vi "首页设置.vi"() -> ()   [LabVIEW 2016]
uses:
  <vilib>/Utility/config.llb/NI_LVConfig.lvlib
panel:
  in  "关闭":bool
  in  "底部状态栏显示信息":string="一体化微型水质监测系统"
  in  "流速":bool caption="氨氮禁用"
  in  "瞬时流量":bool caption="氨氮禁用"
  in  "湿度":bool=TRUE caption="氨氮禁用"
  in  "水位":bool caption="氨氮禁用"
  in  "室温":bool=TRUE caption="氨氮禁用"
  in  "CODCr":bool caption="氨氮禁用"
  in  "CODMn":bool caption="氨氮禁用"
  in  "总氮":bool caption="氨氮禁用"
  in  "总磷":bool caption="氨氮禁用"
  in  "氨氮":bool caption="氨氮禁用"
  in  "Turb":bool caption="氨氮禁用"
  in  "Cond":bool caption="氨氮禁用"
  in  "DO":bool caption="氨氮禁用"
  in  "pH":bool caption="氨氮禁用"
  in  "水温":bool caption="氨氮禁用"
  # "首页显示信息设置"
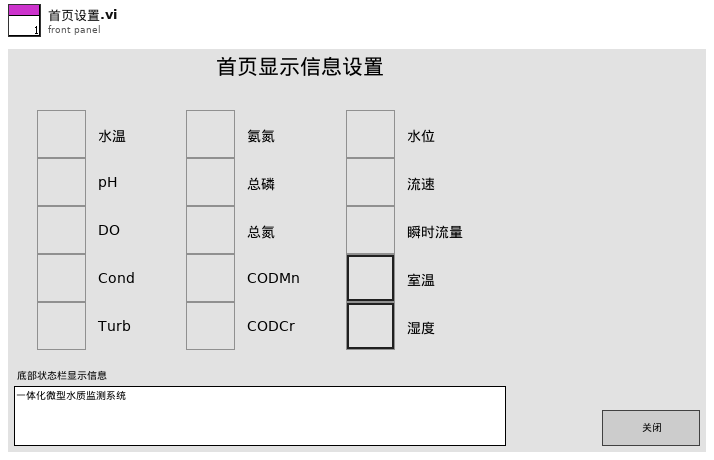
[diagram p1: front panel]
types:
  T1 = typedef "NI_LVConfig.lvlib/Config Data RefNum.ctl" = refnum<k1>
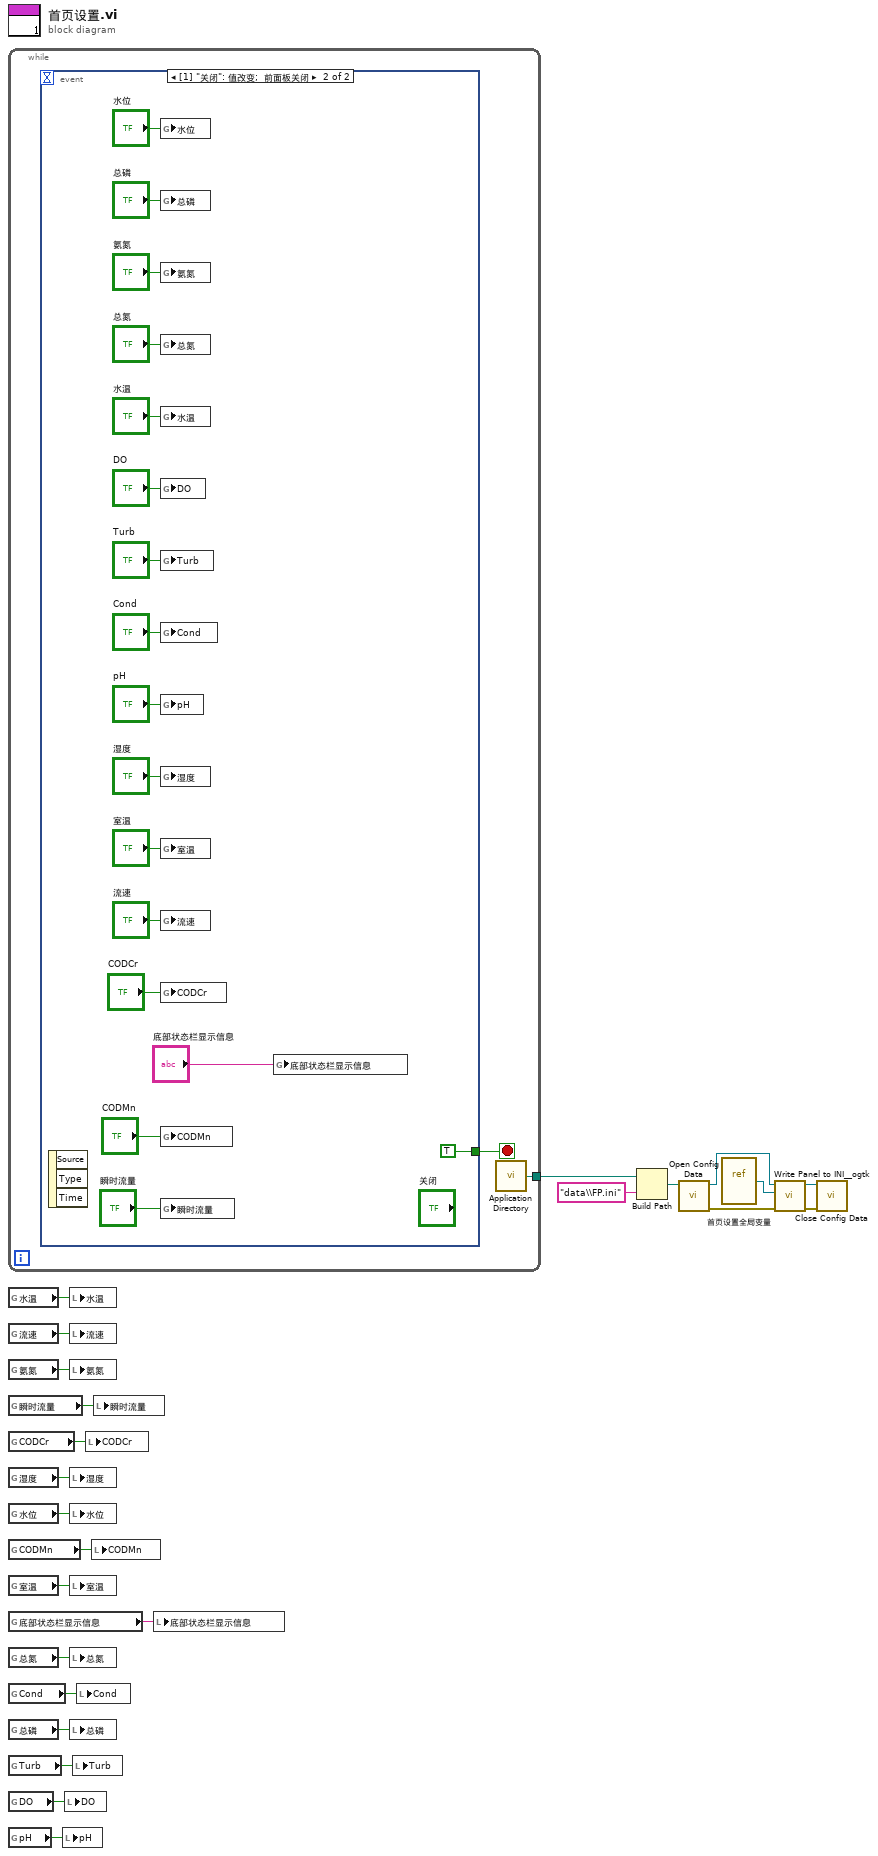
[diagram p0: block diagram]
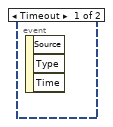
[diagram p2: hidden frame]
diagram:
  n1 = while {
    tunnel: [w25] -> w17
    stop <- w26 stop-if-true
    n2 = event shown="[1] \"关闭\": 值改变;  前面板关闭" {
      selector: _ -> [_ _]
      dyn-events: _ -> [_ _]
      timeout: _ -> [_ _]
      tunnel: [_ TRUE] -> w26
      event Timeout {
        n3 = event-data() -> ()  [unwired: 1 in, 3 out]
      }
      event "关闭": Value Change; Panel Close {
        n4 = event-data() -> ()  [unwired: 1 in, 3 out]
        n5 = global write "首页设置全局变量.vi" "水位"("水位") -> ()
        n6 = global write "首页设置全局变量.vi" "总磷"("总磷") -> ()
        n7 = global write "首页设置全局变量.vi" "氨氮"("氨氮") -> ()
        n8 = global write "首页设置全局变量.vi" "总氮"("总氮") -> ()
        n9 = global write "首页设置全局变量.vi" "水温"("水温") -> ()
        n10 = global write "首页设置全局变量.vi" "DO"("DO") -> ()
        n11 = global write "首页设置全局变量.vi" "Turb"("Turb") -> ()
        n12 = global write "首页设置全局变量.vi" "Cond"("Cond") -> ()
        n13 = global write "首页设置全局变量.vi" "pH"("pH") -> ()
        n14 = global write "首页设置全局变量.vi" "湿度"("湿度") -> ()
        n15 = global write "首页设置全局变量.vi" "室温"("室温") -> ()
        n16 = global write "首页设置全局变量.vi" "流速"("流速") -> ()
        n17 = global write "首页设置全局变量.vi" "CODCr"("CODCr") -> ()
        n18 = global write "首页设置全局变量.vi" "CODMn"("CODMn") -> ()
        n19 = global write "首页设置全局变量.vi" "瞬时流量"("瞬时流量") -> ()
        n20 = global write "首页设置全局变量.vi" "底部状态栏显示信息"("底部状态栏显示信息") -> ()
      }
    }
    n21 = call <vilib>:"Application Directory.vi"() -> ("Application Directory"=w25:path)
  }
  n22 = global read "首页设置全局变量.vi" "水温"() -> (w1:bool)
  n23 = global read "首页设置全局变量.vi" "流速"() -> (w2:bool)
  n24 = global read "首页设置全局变量.vi" "氨氮"() -> (w3:bool)
  n25 = global read "首页设置全局变量.vi" "瞬时流量"() -> (w4:bool)
  n26 = global read "首页设置全局变量.vi" "CODCr"() -> (w5:bool)
  n27 = global read "首页设置全局变量.vi" "湿度"() -> (w6:bool)
  n28 = global read "首页设置全局变量.vi" "水位"() -> (w7:bool)
  n29 = global read "首页设置全局变量.vi" "CODMn"() -> (w8:bool)
  n30 = global read "首页设置全局变量.vi" "室温"() -> (w9:bool)
  n31 = global read "首页设置全局变量.vi" "底部状态栏显示信息"() -> (w10:string)
  n32 = global read "首页设置全局变量.vi" "总氮"() -> (w11:bool)
  n33 = global read "首页设置全局变量.vi" "Cond"() -> (w12:bool)
  n34 = global read "首页设置全局变量.vi" "总磷"() -> (w13:bool)
  n35 = global read "首页设置全局变量.vi" "Turb"() -> (w14:bool)
  n36 = global read "首页设置全局变量.vi" "DO"() -> (w15:bool)
  n37 = global read "首页设置全局变量.vi" "pH"() -> (w16:bool)
  n38 = local write "pH"(w16) -> ()
  n39 = local write "DO"(w15) -> ()
  n40 = local write "水温"(w1) -> ()
  n41 = local write "流速"(w2) -> ()
  n42 = local write "氨氮"(w3) -> ()
  n43 = local write "湿度"(w6) -> ()
  n44 = local write "水位"(w7) -> ()
  n45 = local write "室温"(w9) -> ()
  n46 = local write "总氮"(w11) -> ()
  n47 = local write "总磷"(w13) -> ()
  n48 = local write "Turb"(w14) -> ()
  n49 = local write "Cond"(w12) -> ()
  n50 = local write "CODCr"(w5) -> ()
  n51 = local write "CODMn"(w8) -> ()
  n52 = local write "瞬时流量"(w4) -> ()
  n53 = local write "底部状态栏显示信息"(w10) -> ()
  n54 = Build Path(base path=w17, name or relative path="data\\FP.ini" ("名称或相对路径")) -> (appended path=w19:path)
  n55 = call <vilib>:"Open Config Data.vi"("configuration file path"=w19) -> ("error out"=w23:errorcluster, "refnum"=w20:T1)  [unwired: 8 in, 1 out]
  n56 = vi-ref "首页设置全局变量.vi"() -> (w21:refnum<vi>)
  n57 = call <userlib>:"Write Panel to INI__ogtk.vi"("error in (no error)"=w23, "VI ref"=w21, "refnum"=w20) -> ("error out"=w24:errorcluster, "refnum out"=w22:T1)  [unwired: 7 in]
  n58 = call <vilib>:"Close Config Data.vi"("error in (no error)"=w24, "refnum"=w22) -> ()  [unwired: 8 in, 2 out]
